vi "hello world.vi"   [LabVIEW 2017]
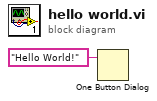
[diagram p0: block diagram]
diagram:
  n1 = One Button Dialog(message="Hello World!") -> ()  [unwired: 1 in, 1 out]
